vi "Get Sheet Names.vi"(8 "error in":errorcluster, 11 "SpreadsheetDoc in":refnum<k24>) -> (0 "error out":errorcluster, 2 "Sheet Names":string[](array[string]), 3 "SpreadsheetDoc out":refnum<k24>)   [LabVIEW 2019, in "Open Xml.lvlib"]
uses:
  Open Xml.lvlib
  D:/git/Open-Xml-LabVIEW/Source/DocumentFormat.OpenXml.Framework.dll
  DocumentFormat.OpenXml.Framework.dll
  D:/git/Open-Xml-LabVIEW/Source/DocumentFormat.OpenXml.dll
  DocumentFormat.OpenXml.dll
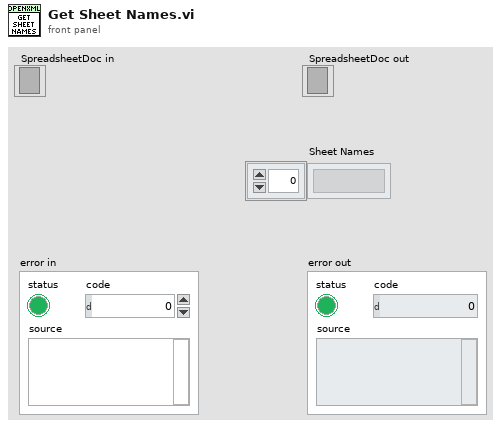
[diagram p1: front panel]
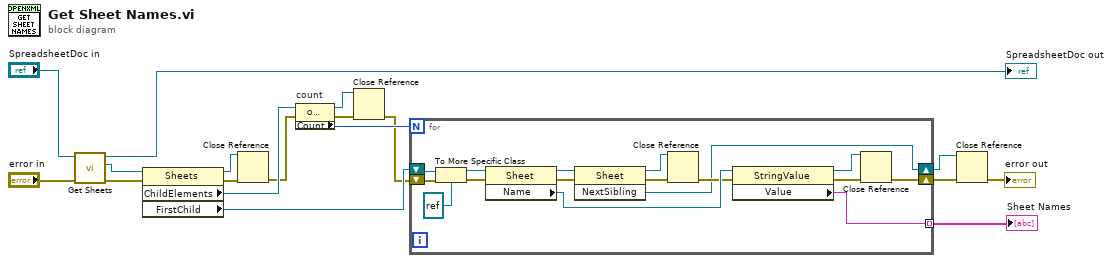
[diagram p0: block diagram]
diagram:
  n1 = call "Get Sheets.vi"("error in"="error in", "SpreadsheetDocument in"="SpreadsheetDoc in") -> ("error out"=w15:errorcluster, "Sheets"=w14:refnum<k24>, "SpreadsheetDocument out"=→"SpreadsheetDoc out":refnum<k24>)  [unwired: 7 in]
  n2 = property class="Sheets"(reference=w14, error in=w15) -> (reference out=w7:refnum<k24>, error out=w6:errorcluster, "ChildElements"=w13:refnum<k24>, "FirstChild"=w11:refnum<k24>)
  n3 = Close Reference(reference=w7, error in (no error)=w6) -> (error out=w5:errorcluster)
  n4 = property on="count" class="OpenXmlElementList"(reference=w13, error in=w5) -> (reference out=w8:refnum<k24>, error out=w4:errorcluster, "Count"=w12:i32)
  n5 = Close Reference(reference=w8, error in (no error)=w4) -> (error out=w3:errorcluster)
  n6 = for {
    N: w12 -> [_]
    shift-right: [w25] -> w10
    shift-left: w3 -> [w34]
    tunnel: [w26] -> w9 mode=indexing
    shift-right: [w19] -> w1
    shift-left: w11 -> [w33]
    n7 = To More Specific Class(target class=refnum<k24> refnum ("FirstChild"), reference=w33, error in=w34) -> (specific class reference=w29:refnum<k24>, error out=w31:errorcluster)
    n8 = property class="Sheet"(reference=w29, error in=w31) -> (reference out=w21:refnum<k24>, error out=w30:errorcluster, "Name"=w27:refnum<k24>)
    n9 = invoke class="Sheet" method="NextSibling"(reference=w21, error in=w30) -> (reference out=w20:refnum<k24>, error out=w22:errorcluster, "NextSibling"=w19:refnum<k24>)  [unwired: 1 in]
    n10 = Close Reference(reference=w20, error in (no error)=w22) -> (error out=w23:errorcluster)
    n11 = property class="StringValue"(reference=w27, error in=w23) -> (reference out=w24:refnum<k24>, error out=w28:errorcluster, "Value"=w26:string)
    n12 = Close Reference(reference=w24, error in (no error)=w28) -> (error out=w25:errorcluster)
  }
  "Sheet Names" <- w9
  n13 = Close Reference(reference=w1, error in (no error)=w10) -> (error out=→"error out":errorcluster)
